vi "WriteConfigFile.vi"(8 "ErrorIn":errorcluster, 10 "RTConfig":T1, 11 "configuration file path":path) -> (0 "ErrorOut":errorcluster)   [LabVIEW 2018]
doc: "Write the configuration (INI) file specified in ClusterIn.Paths.CfgFile. Add elements to this VI for each cluster element that you wish to save.\n\nCopyright © 2011 Epimedia, Inc. All Rights Reserved.\n\nThe Epimedia Application Library is Copyright © 2009-2011 Epimedia, Inc. \nAll Rights Reserved. Used under license."
uses:
  Controls/RT_Config.ctl
  <vilib>/Utility/config.llb/Write Key (String).vi
  <vilib>/Utility/config.llb/Write Key (Double).vi
  <vilib>/Utility/config.llb/NI_LVConfig.lvlib
panel:
  # "Copyright © 2011 Epimedia, Inc. All Rights Reserved.\n\nThe Epimedia Application Library is Copyright © 2009-2011 Epimedia, Inc. \nAll Rights Reserved. Used under license."
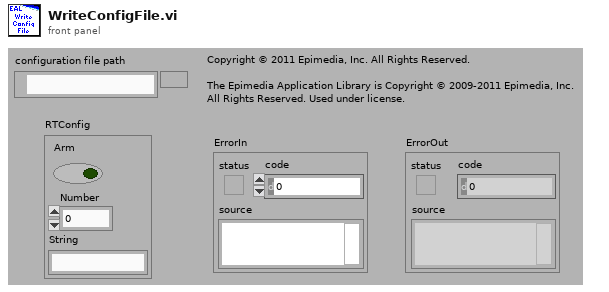
[diagram p1: front panel]
types:
  T1 = typedef "RT_Config.ctl" = cluster{"Arm":bool, "Number":dbl, "String":string}
  T2 = typedef "NI_LVConfig.lvlib/Config Data RefNum.ctl" = refnum<k1>
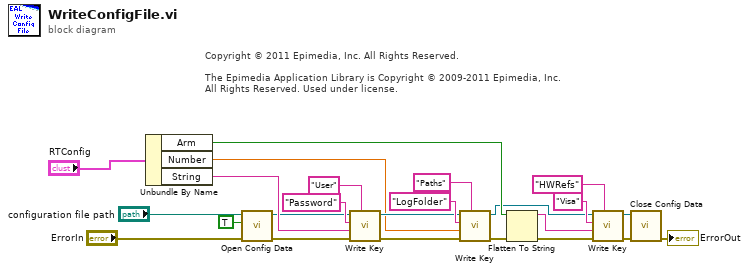
[diagram p0: block diagram]
diagram:
  # "Copyright © 2011 Epimedia, Inc. All Rights Reserved.\n\nThe Epimedia Application Library is Copyright © 2009-2011 Epimedia, Inc. \nAll Rights Reserved. Used under license."
  n1 = Unbundle By Name("RTConfig") -> ("Arm"=w9:bool, "Number"=w10:dbl, "String"=w18:string)
  n2 = call <vilib>:"Open Config Data.vi"("error in (no error)"="ErrorIn", "create file if necessary (T)"=TRUE ("create file if necessary? (T)"), "configuration file path"="configuration file path") -> ("error out"=w14:errorcluster, "refnum"=w15:T2)  [unwired: 6 in, 1 out]
  n3 = call-poly <vilib>:"Write Key.vi"("section"="User" ("key"), "error in (no error)"=w14, "value"=w18, "key"="Password", "refnum"=w15) -> ("error out"=w11:errorcluster, "refnum out"=w12:T2)  [unwired: 1 in, 4 out]
  n4 = call-poly <vilib>:"Write Key.vi"("section"="Paths" ("key"), "error in (no error)"=w11, "value"=w10, "key"="LogFolder", "refnum"=w12) -> ("error out"=w7:errorcluster, "refnum out"=w8:T2)  [unwired: 3 in, 2 out]
  n5 = Flatten To String(anything=w9, error in (no error)=w7) -> (data string=w5:string, error out=w6:errorcluster)  [unwired: 2 in, 1 out]
  n6 = call-poly <vilib>:"Write Key.vi"("section"="HWRefs" ("key"), "error in (no error)"=w6, "value"=w5, "key"="Visa", "refnum"=w8) -> ("error out"=w3:errorcluster, "refnum out"=w4:T2)  [unwired: 1 in, 4 out]
  n7 = call <vilib>:"Close Config Data.vi"("error in (no error)"=w3, "refnum"=w4) -> ("error out"=→"ErrorOut":errorcluster)  [unwired: 1 in, 8 out]
